vi "Voltage - Finite Input.vi"() -> ()   [LabVIEW 2014]
doc: "This example demonstrates how to acquire a single buffer of voltage measurements using a DAQmx device.\n\nFor instructions on how to connect your signals to the DAQ device, refer to your device documentation."
uses:
  <vilib>/Utility/error.llb/DialogType.ctl
  <vilib>/DAQmx/create/channels.llb/DAQmx Create Channel (AI-Voltage-Basic).vi
  <vilib>/DAQmx/configure/timing.llb/DAQmx Timing (Sample Clock).vi
  <vilib>/DAQmx/read.llb/DAQmx Read (Analog 1D Wfm NChan NSamp).vi
panel:
  out "Waveform Graph":waveform(dbl)[](graph)
  in  "Number of Samples":i32=100
  in  "Sample Rate":dbl=1000.0
  in  "Sample Clock Source":tag="OnboardClock"
  in  "Terminal Configuration":i32(ring)=-1 items=["default"=-1, "RSE"=10083, "NRSE"=10078, "Differential"=10106, "Pseudodifferential"=12529]
  in  "Max Voltage":dbl=5.0
  in  "Min Voltage":dbl=-5.0
  in  "Physical Channel":tag="Dev1/ai0"
  # "Channel Settings"
  # "Acquired Data"
  # "Timing Settings"
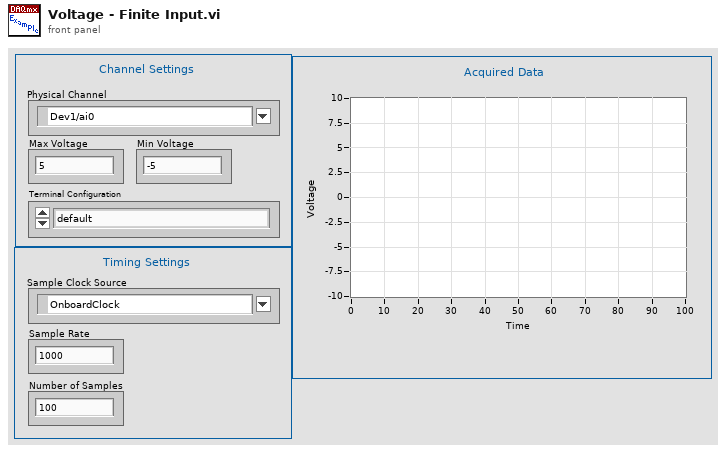
[diagram p1: front panel]
types:
  T1 = typedef "DialogType.ctl" = u16
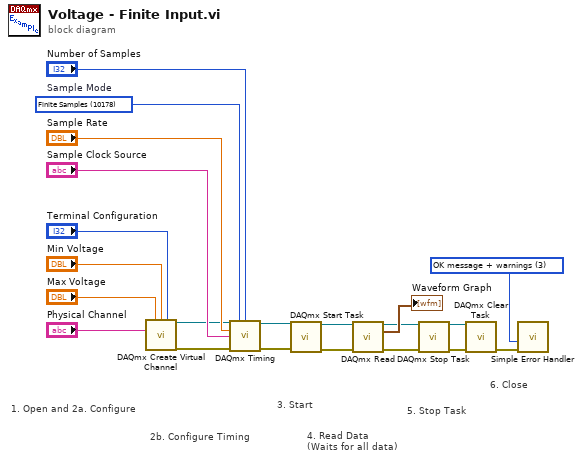
[diagram p0: block diagram]
diagram:
  w4 = T1 3 items=["no dialog", "OK message", "continue or stop message", "OK message + warnings", "continue/stop + warnings"] ("type of dialog (OK msg:1)")
  w21 = 10178 items=["Finite Samples"=10178, "Continuous Samples"=10123, "Hardware Timed Single Point"=12522]  # Sample Mode
  # "2b. Configure Timing"
  # "6. Close"
  # "5. Stop Task"
  # "3. Start"
  # "4. Read Data\n(Waits for all data)"
  # "1. Open and 2a. Configure"
  n1 = call-poly <vilib>:"DAQmx Create Virtual Channel.vi"("maximum value"="Max Voltage", "minimum value"="Min Voltage", "input terminal configuration"="Terminal Configuration", "physical channels"="Physical Channel") -> ("task out"=w3:refnum<k21>, "error out"=w20:errorcluster)  [unwired: 10 in]
  n2 = call-poly <vilib>:"DAQmx Timing.vi"("task/channels in"=w3, "sample mode"=w21, "samples per channel"="Number of Samples", "rate"="Sample Rate", "source"="Sample Clock Source", "error in"=w20) -> ("task out"=w2:refnum<k21>, "error out"=w1:errorcluster)  [unwired: 8 in]
  n3 = call <vilib>:"DAQmx Start Task.vi"("task/channels in"=w2, "error in"=w1) -> ("task out"=w19:refnum<k21>, "error out"=w18:errorcluster)  [unwired: 12 in]
  n4 = call-poly <vilib>:"DAQmx Read.vi"("task/channels in"=w19, "error in"=w18) -> ("task out"=w6:refnum<k21>, "data"=→"Waveform Graph":waveform(dbl)[], "error out"=w5:errorcluster)  [unwired: 11 in]
  n5 = call <vilib>:"DAQmx Stop Task.vi"("task/channels in"=w6, "error in"=w5) -> ("task out"=w8:refnum<k21>, "error out"=w7:errorcluster)  [unwired: 12 in]
  n6 = call <vilib>:"DAQmx Clear Task.vi"("task in"=w8, "error in"=w7) -> ("error out"=w17:errorcluster)  [unwired: 13 in]
  n7 = call <vilib>:"Simple Error Handler.vi"("type of dialog (OK msg:1)"=w4, "error in (no error)"=w17) -> ()  [unwired: 3 in, 5 out]
